vi "Configure RT Phase Noise Impairment.vi"(4 "Stop Frequency (30 kHz)":dbl=30000.0, 6 "Start Frequency (1 kHz)":dbl=1000.0, 7 "Enable Phase Noise Impairment (F:Disable)":bool, 8 "error in (no error)":errorcluster, 9 "Flat Amplitude (-70 dBc/Hz)":dbl=-70.0, 10 "Modulation Format (1: Dual Modulation)":u16(ring)=1 items=["Dual Modulation"=1, "Dual ARB"=2, "Multitone"=3, "Phase Noise"=5, "Two-tone"=6], 11 "VISA resource name":refnum<visa-resource-name>) -> (0 "error out":errorcluster, 3 "VISA resource name out":refnum<visa-resource-name>)   [LabVIEW 2011, in "Agilent PSG MXG Series.lvlib"]
doc: "Configures the phase noise impairment.\n\n<B>Notes:</B>\n(1) This VI is valid only in N5182A that installs <B>Option 651</B> or <B>Option 652</B> or <B>Option 654</B> (Internal baseband generator), and <B>Option 432</B> (Phase noise impairment)."
uses:
  Agilent PSG MXG Series.lvlib
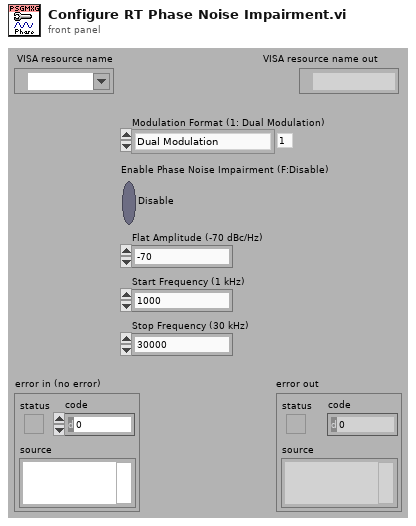
[diagram p1: front panel]
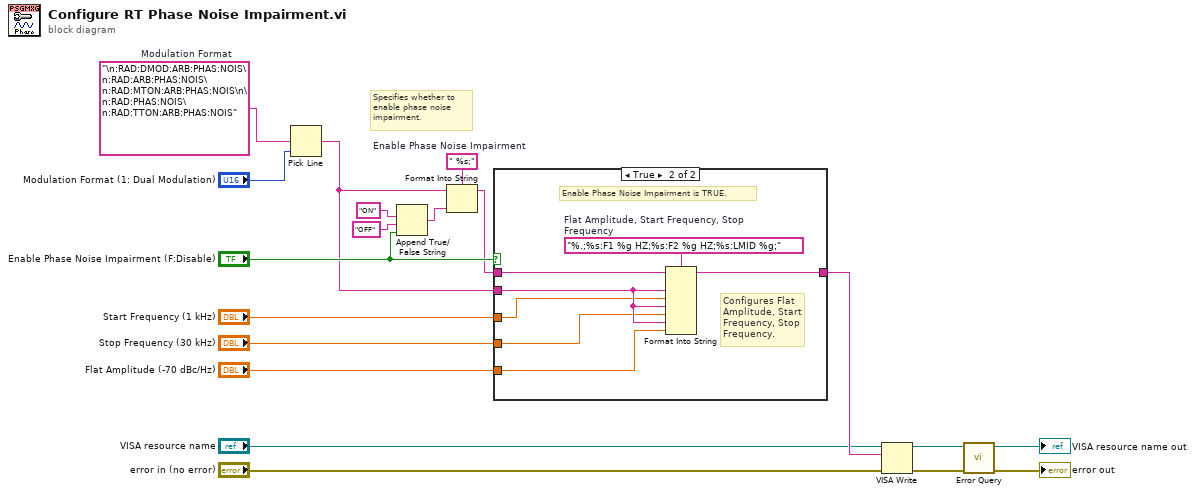
[diagram p0: block diagram]
diagram:
  w17 = " %s;"  # Enable Phase Noise Impairment
  w18 = "\n:RAD:DMOD:ARB:PHAS:NOIS\n:RAD:ARB:PHAS:NOIS\n:RAD:MTON:ARB:PHAS:NOIS\n\n:RAD:PHAS:NOIS\n:RAD:TTON:ARB:PHAS:NOIS"  # Modulation Format
  # "Specifies whether to\nenable phase noise\nimpairment."
  n1 = Pick Line(multi-line string=w18, line index="Modulation Format (1: Dual Modulation)") -> (output string=w12:string)  [unwired: 1 in]
  n2 = Append True/False String(1:"Enable Phase Noise Impairment (F:Disable)", 2:"OFF" ("false string"), 3:"ON" ("true string")) -> (0:w16:string)  [unwired: 1 in]
  n3 = Format Into String(format string=w17, initial string=w12, w16) -> (resulting string=w8:string)  [unwired: 1 in, 1 out]
  n4 = case shown="True" "Enable Phase Noise Impairment (F:Disable)" {
    tunnel: w12 -> [_ w26]
    tunnel: "Flat Amplitude (-70 dBc/Hz)" -> [_ w21]
    tunnel: "Start Frequency (1 kHz)" -> [_ w23]
    tunnel: "Stop Frequency (30 kHz)" -> [_ w22]
    tunnel: w8 -> [w20 w25]
    tunnel: [w20 w24] -> w5
    frame False {
      # "Enable Phase Noise Impairment is FALSE."
    }
    frame True {
      w27 = "%.;%s:F1 %g HZ;%s:F2 %g HZ;%s:LMID %g;"  # Flat Amplitude, Start Frequency, Stop Frequency
      # "Configures Flat\nAmplitude, Start\nFrequency, Stop\nFrequency."
      # "Enable Phase Noise Impairment is TRUE."
      n5 = Format Into String(format string=w27, initial string=w25, w26, w23, w26, w22, w26, w21) -> (resulting string=w24:string)  [unwired: 1 in, 1 out]
    }
  }
  n6 = VISA Write(VISA resource name="VISA resource name", write buffer=w5, error in (no error)="error in (no error)") -> (VISA resource name out=w7:refnum<visa-resource-name>, error out=w6:errorcluster)  [unwired: 1 out]
  n7 = call "Error Query.vi"("error in (no error)"=w6, "VISA resource name"=w7) -> ("error out"=→"error out":errorcluster, "VISA resource name out"=→"VISA resource name out":refnum<visa-resource-name>)  [unwired: 6 in, 2 out]
